vi "Min Panel Size.vi"(8 "error in (no error)":errorcluster) -> (0 "error out":errorcluster, 3 "Static out":refnum<class "Absolute Size.lvclass">)   [LabVIEW 2019, in "Panel.lvlib" / "Absolute Size.lvclass"]
doc: "Sets the size of the panel to the Min Panel Size of the shown front panel. If no Min Panel Size is set then the panel size will be unchanged.\n\n<B>Error In:</B> Describes error conditions that occur before this node runs.\n\n<B>Static Out:</B> Absolute Size object.\n<B>Error Out:</B> Contains error information.\n----\nPlease see the following web address for additional documentation and tutorial information:\nhttp://www.mooregoodideas.com/mgi-panel-manager/\n\nAuthor: Derek Trepanier\n\nCopyright (c) 2018, Moore Good Ideas, Inc.\n\nAll rights reserved.\n\nRedistribution and use in source and binary forms, with or without modification, are permitted provided that the following conditions are met:\n\n * Redistributions of source code must retain the above copyright notice, this list of conditions and the following disclaimer.\n * Redistributions in binary form must reproduce the above copyright notice, this list of conditions and the following disclaimer in the documentation and/or other materials provided with the distribution.\n * Neither the name of Moore Good Ideas, Inc. nor the names of its contributors may be used to endorse or promote products derived from this software without specific prior written permission.\n\nTHIS SOFTWARE IS PROVIDED BY THE COPYRIGHT HOLDERS AND CONTRIBUTORS \"AS IS\" AND ANY EXPRESS OR IMPLIED WARRANTIES, INCLUDING, BUT NOT LIMITED TO, THE IMPLIED WARRANTIES OF MERCHANTABILITY AND FITNESS FOR A PARTICULAR PURPOSE ARE DISCLAIMED. IN NO EVENT SHALL THE COPYRIGHT OWNER OR CONTRIBUTORS BE LIABLE FOR ANY DIRECT, INDIRECT, INCIDENTAL, SPECIAL, EXEMPLARY, OR CONSEQUENTIAL DAMAGES (INCLUDING, BUT NOT LIMITED TO, PROCUREMENT OF SUBSTITUTE GOODS OR SERVICES; LOSS OF USE, DATA, OR PROFITS; OR BUSINESS INTERRUPTION) HOWEVER CAUSED AND ON ANY THEORY OF LIABILITY, WHETHER IN CONTRACT, STRICT LIABILITY, OR TORT (INCLUDING NEGLIGENCE OR OTHERWISE) ARISING IN ANY WAY OUT OF THE USE OF THIS SOFTWARE, EVEN IF ADVISED OF THE POSSIBILITY OF SUCH DAMAGE."
uses:
  Absolute Size.lvclass
  Absolute Size.lvclass/Absolute Size.ctl
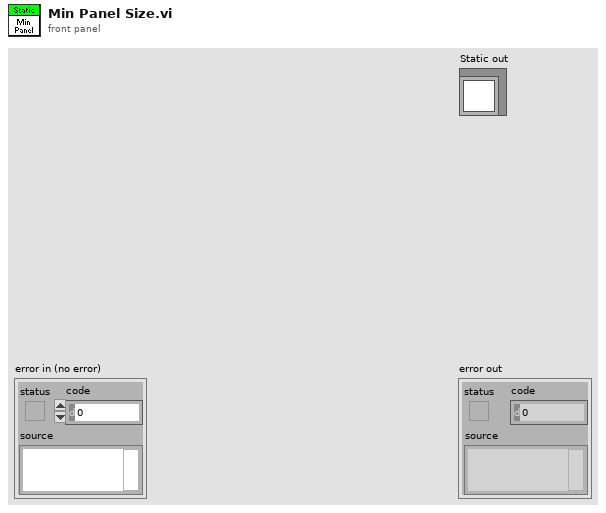
[diagram p1: front panel]
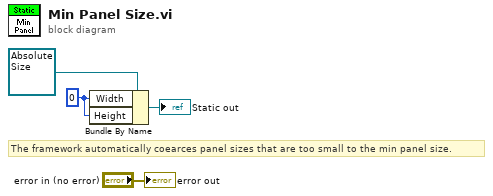
[diagram p0: block diagram]
diagram:
  w1 = i16 0 ("Width")
  # "The framework automatically coearces panel sizes that are too small to the min panel size."
  n1 = Bundle By Name(cluster=refnum<class "Absolute Size.lvclass"> refnum ("Static in"), "Width"=w1, "Height"=w1) -> (→"Static out":refnum<class "Absolute Size.lvclass">)
  "error out" <- "error in (no error)"
